vi "ComputeCircleROI.vi"(1 "Circles":T2(array[cluster])) -> (0 "Rectangle":T1 {"Rotation" min=-90.0 max=90.0 step=1.0 format="%.2f"; "Left" scale=0.0..1024.0; "Right" scale=0.0..1024.0})   [LabVIEW 2017]
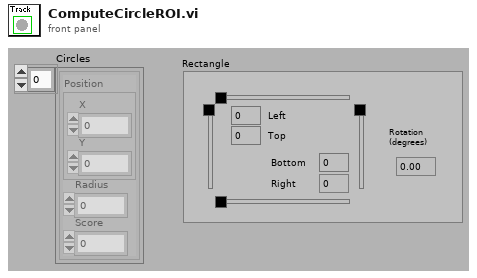
[diagram p1: front panel]
types:
  T1 = typedef "IMAQ Rectangle" = cluster{"Left":i32, "Top":i32, "Right":i32, "Bottom":i32, "Rotation":dbl}
  T2 = cluster{"Position":cluster{"X":sgl, "Y":sgl}, "Radius":dbl, "Score":dbl}[]
  T3 = cluster{"Position":cluster{"X":sgl, "Y":sgl}, "Radius":dbl, "Score":dbl}
  T4 = cluster{"X":dbl, "Y":dbl, "X":dbl, "Y":dbl, "y":dbl}
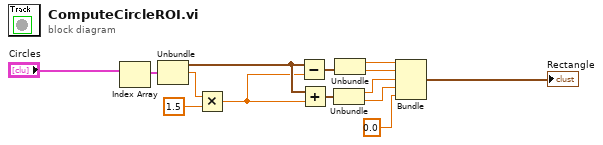
[diagram p0: block diagram]
diagram:
  n1 = Index Array(array="Circles") -> (element=w14:T3)  [unwired: 1 in]
  n2 = Unbundle(w14) -> ("Position"=w5:cluster{"X":sgl, "Y":sgl}, "Radius"=w4:dbl)  [unwired: 1 out]
  n3 = Multiply(x=w4, y=1.5) -> (x*y=w2:dbl)
  n4 = Subtract(x=w5, y=w2) -> (x-y=w12:cluster{"X":dbl, "Y":dbl})
  n5 = Add(x=w5, y=w2) -> (x+y=w11:cluster{"X":dbl, "Y":dbl})
  n6 = Unbundle(w11) -> ("X"=w8:dbl, "Y"=w7:dbl)
  n7 = Unbundle(w12) -> ("X"=w10:dbl, "Y"=w9:dbl)
  n8 = Bundle("X"=w10, "Y"=w9, "X"=w8, "Y"=w7, "y"=0.0) -> (→"Rectangle":T4)  [unwired: 1 in]
